vi "Lakeshore-temp-control.vi"(8 "Sample Channel Units":u16(ring) items=["Kelvin", "Celsius", "Sensor Units"], 9 "Setpoint (0.0000)":dbl=20.0 min=-273.0 max=999.9999 step=0.0001 format="%.4f", 10 "Sample Channels":u16(ring) items=["Sensor A", "Sensor B"], 11 "VISA Resource Name":refnum<visa-resource-name>="GPIB0::12::INSTR") -> (0 "Heater Output":i32(slide) min=0 max=100 step=1 scale=0.0..100.0, 1 "Temp. Setpoint (0.0000)":dbl=20.0 min=-273.0 max=999.9999 step=0.0001 format="%.4f", 2 "Sample Channel Unit":u16(ring), 3 "Sample Sensor Data":dbl min=-273.0 max=999.0 step=0.0001 format="%.4f", 5 "Sample Channel":u16(ring) items=["Sensor A", "Sensor B"])   [LabVIEW 2009]
panel:
  out "Tab Control":enum32{"Autotune", "Manual PID"}(tab)=enum."Manual PID"
  in  "Autotune":u16(ring)=3 items=["AutoTune P"=1, "AutoTune PI"=2, "AutoTune PID"=3, "Zone"=4]
  in  "PID":cluster{"P":dbl, "I":dbl, "D":dbl}={"P"=55.0, "I"=15.0, "D"=2.0}
  in  "Autotuning Status":enum32{"Auto Tune", "Manual"}(radio)=enum."Manual"
  in  "stop":bool
  in  "Heater Range (0: Off)":u16(ring) items=["Off", "Low (0.1 A)", "Med (0.3 A)", "High (1.0 A)"]
  # "330 LakeShore Temperature Controller"
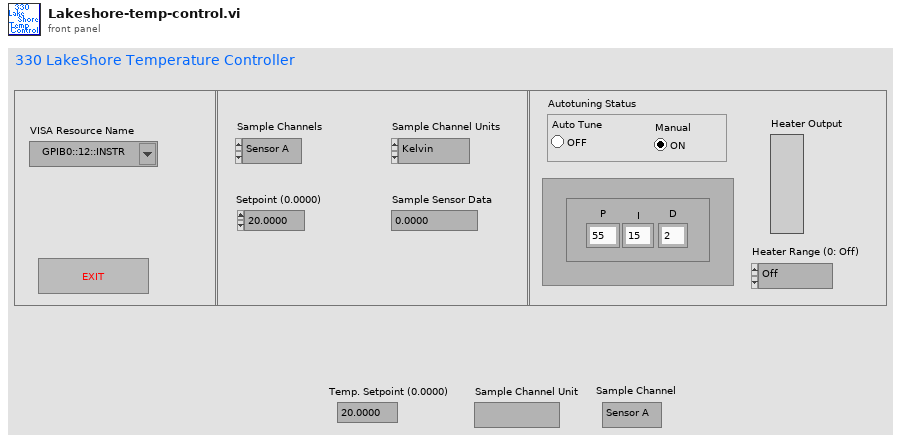
[diagram p1: front panel]
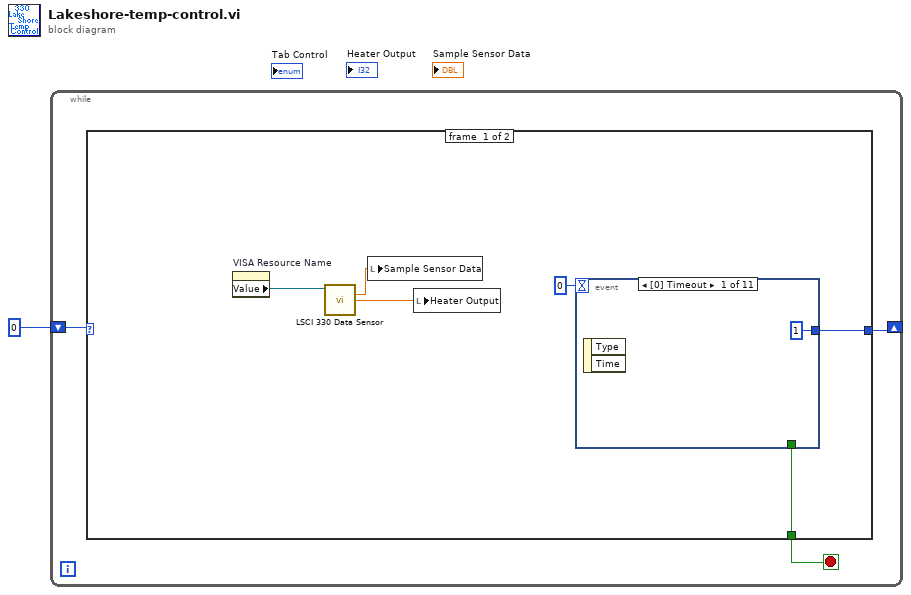
[diagram p0: block diagram]
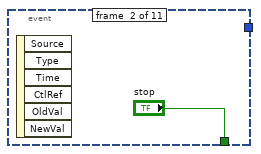
[diagram p2: hidden frame]
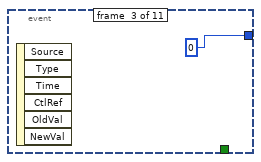
[diagram p3: hidden frame]
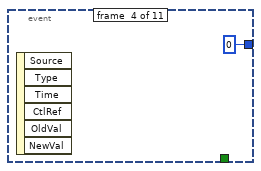
[diagram p4: hidden frame]
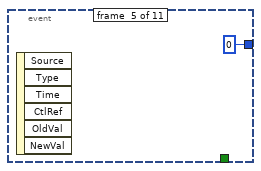
[diagram p5: hidden frame]
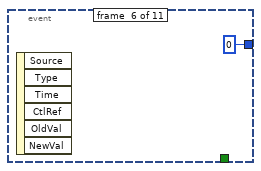
[diagram p6: hidden frame]
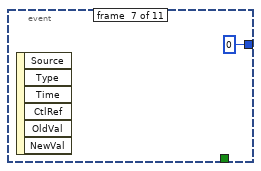
[diagram p7: hidden frame]
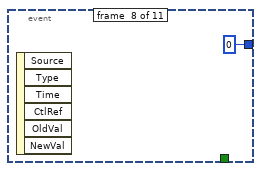
[diagram p8: hidden frame]
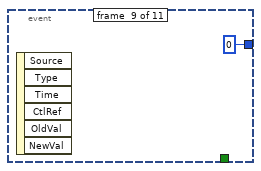
[diagram p9: hidden frame]
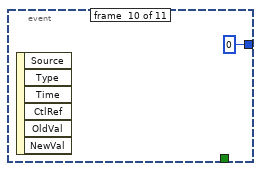
[diagram p10: hidden frame]
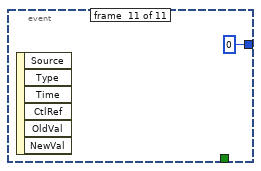
[diagram p11: hidden frame]
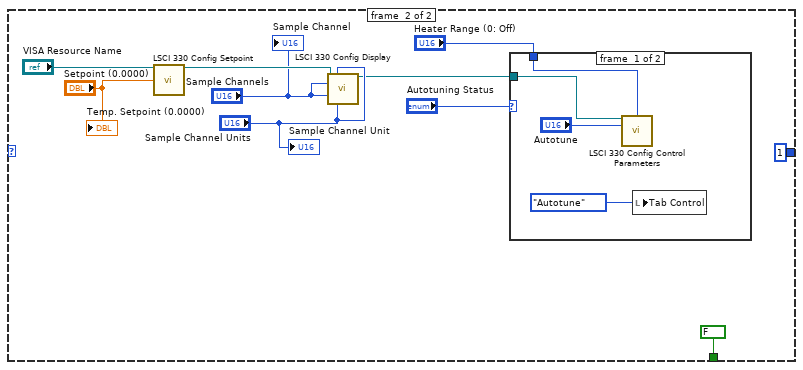
[diagram p12: hidden frame]
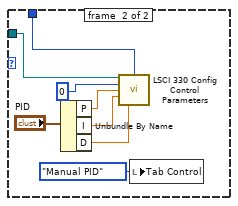
[diagram p13: hidden frame]
diagram:
  n1 = while {
    shift-right: [w3] -> _
    shift-left: 0 -> [w4]
    stop <- w2 stop-if-true
    n2 = case shown="1, Default" w4 {
      tunnel: [w7 1] -> w3
      tunnel: [w6 FALSE ("stop")] -> w2
      frame #0 {
        n3 = property on="VISA Resource Name" class="VISAName"() -> ("Value"=w9:refnum<visa-resource-name>)  [unwired: 2 in, 2 out]
        n4 = call "LSCI 330 Data Sensor.vi"("VISA session"=w9) -> ("Sample Sensor Data"=w10:dbl, "Control Sensor Data"=w5:dbl)  [unwired: 11 in, 2 out]
        n5 = local write "Sample Sensor Data"(w10) -> ()
        n6 = local write "Heater Output"(w5) -> ()
        n7 = event shown="[0] Timeout" {
          selector: _ -> [_ _ _ _ _ _ _ _ _ _ _]
          dyn-events: _ -> [_ _ _ _ _ _ _ _ _ _ _]
          timeout: 0 -> [_ _ _ _ _ _ _ _ _ _ _]
          tunnel: [1 _ 0 0 0 0 0 0 0 0 0] -> w7
          tunnel: [_ "stop" _ _ _ _ _ _ _ _ _] -> w6
          event #0 {
            n8 = event-data() -> ()  [unwired: 1 in, 2 out]
          }
          event #1 {
            n9 = event-data() -> ()  [unwired: 1 in, 6 out]
          }
          event #2 {
            n10 = event-data() -> ()  [unwired: 1 in, 6 out]
          }
          event #3 {
            n11 = event-data() -> ()  [unwired: 1 in, 6 out]
          }
          event #4 {
            n12 = event-data() -> ()  [unwired: 1 in, 6 out]
          }
          event #5 {
            n13 = event-data() -> ()  [unwired: 1 in, 6 out]
          }
          event #6 {
            n14 = event-data() -> ()  [unwired: 1 in, 6 out]
          }
          event #7 {
            n15 = event-data() -> ()  [unwired: 1 in, 6 out]
          }
          event #8 {
            n16 = event-data() -> ()  [unwired: 1 in, 6 out]
          }
          event #9 {
            n17 = event-data() -> ()  [unwired: 1 in, 6 out]
          }
          event #10 {
            n18 = event-data() -> ()  [unwired: 1 in, 6 out]
          }
        }
      }
      frame #1 {
        n19 = call "LSCI 330 Config Setpoint.vi"("VISA session"="VISA Resource Name", "Setpoint (0.0000)"="Setpoint (0.0000)") -> ("dup VISA session"=w28:refnum<visa-resource-name>)  [unwired: 12 in, 1 out]
        n20 = call "LSCI 330 Config Display.vi"("VISA session"=w28, "Control Channel Units (0: Kelvin)"="Sample Channel Units", "Control Channel (0: Sensor A)"="Sample Channels", "Sample Channel (0: Sensor A)"="Sample Channels", "Sample Channel Units (0: Kelvin)"="Sample Channel Units") -> ("dup VISA session"=w24:refnum<visa-resource-name>)  [unwired: 9 in, 1 out]
        n21 = case shown="\"Manual\", Default" "Autotuning Status" {
          tunnel: w24 -> [w33 w36]
          tunnel: "Heater Range (0: Off)" -> [w32 w37]
          frame #0 {
            n22 = call "LSCI 330 Config Control Parameters.vi"("VISA session"=w33, "Heater Range (0: Off)"=w32, "Autotuning Status (0: Manual PID)"="Autotune") -> ()  [unwired: 11 in, 2 out]
            n23 = local write "Tab Control"(enum32{"Autotune", "Manual PID"}."Autotune" ("Tab Control")) -> ()
          }
          frame #1 {
            n24 = Unbundle By Name("PID") -> ("P"=w40:dbl, "I"=w39:dbl, "D"=w38:dbl)
            n25 = call "LSCI 330 Config Control Parameters.vi"("VISA session"=w36, "Heater Range (0: Off)"=w37, "Autotuning Status (0: Manual PID)"=u16 0, "Gain (P) (0)"=w40, "Reset (I) (0)"=w39, "Rate (D) (0)"=w38) -> ()  [unwired: 8 in, 2 out]
            n26 = local write "Tab Control"(enum32{"Autotune", "Manual PID"}."Manual PID" ("Tab Control")) -> ()
          }
        }
        "Temp. Setpoint (0.0000)" <- "Setpoint (0.0000)"
        "Sample Channel Unit" <- "Sample Channel Units"
        "Sample Channel" <- "Sample Channels"
      }
    }
  }
